vi "Control_Panel_Set.vi"   [LabVIEW 2019]
uses:
  Control_Panel_States.ctl
  Control_Panel_Globals.vi
types:
  T1 = typedef "Control_Panel_States.ctl" = enum16{"No-Op", "Rotational_Control", "Positional_Control", "Manual_Control"}
  T2 = typedef "Control_Panel_Cluster.ctl" = cluster{"Control_State":T1, "Start_Movement":bool, "Abort":bool, "Rotation_Control?":bool, "Positional_Control? ":bool, "Throttle":dbl, "Extend?":bool}
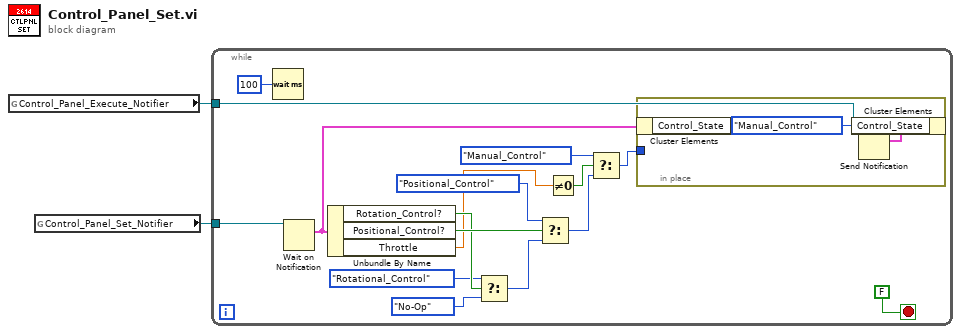
[diagram p0: block diagram]
diagram:
  n1 = global read "Control_Panel_Globals.vi" "Control_Panel_Execute_Notifier"() -> (w1:refnum<notifier>)
  n2 = global read "Control_Panel_Globals.vi" "Control_Panel_Set_Notifier"() -> (w2:refnum<notifier>)
  n3 = while {
    tunnel: w2 -> [w18]
    tunnel: w1 -> [w17]
    stop <- FALSE stop-if-true
    n4 = Wait (ms)(milliseconds to wait=u32 100) -> ()  [unwired: 1 out]
    n5 = Wait on Notification(notifier=w18) -> (notification=w16:T2)  [unwired: 3 in, 3 out]
    n6 = Unbundle By Name(w16) -> ("Rotation_Control?"=w12:bool, "Positional_Control?"=w14:bool, "Throttle"=w3:dbl)
    n7 = Select(t=Control_Panel_States."Rotational_Control" ("Control_State"), s=w12, f=Control_Panel_States."No-Op" ("Control_State")) -> (s? t:f=w13:T1)
    n8 = Select(t=Control_Panel_States."Positional_Control" ("Control_State"), s=w14, f=w13) -> (s? t:f=w9:T1)
    n9 = Not Equal To 0?(x=w3) -> (x != 0?=w4:bool)
    n10 = Select(t=Control_Panel_States."Manual_Control" ("Control_State"), s=w4, f=w9) -> (s? t:f=w8:T1)
    n11 = in-place {
      in-place-border: w8 -> [_]
      n12 = in-place-cluster #1(w16) -> ()  [unwired: 1 out]
      n13 = in-place-cluster #1("Control_State"=Control_Panel_States."Manual_Control") -> (w15:T2)
    }
    n14 = Send Notification(notification=w15, notifier=w17) -> ()  [unwired: 1 in, 2 out]
  }
